vi "API VI Generation tester.vi"() -> ()   [LabVIEW 2020, in "Method Generation.lvlib" / "API VI Generator.lvclass"]
uses:
  API VI Generator.lvclass
  API VI Generator.lvclass/API VI Generator.ctl
panel:
  out "error out":errorcluster
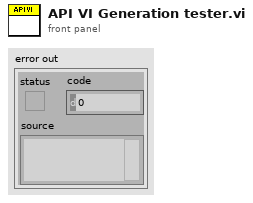
[diagram p1: front panel]
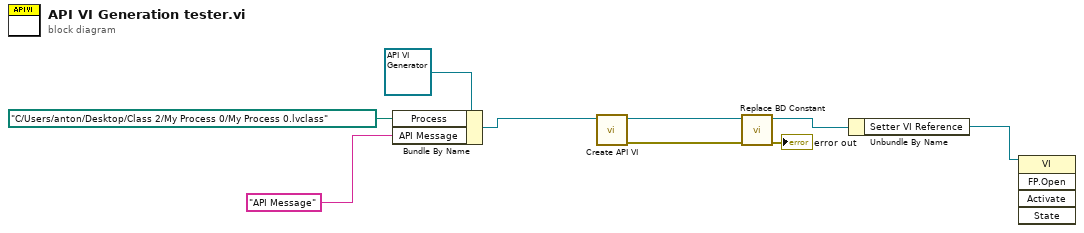
[diagram p0: block diagram]
diagram:
  n1 = Bundle By Name(cluster=refnum<class "API VI Generator.lvclass"> refnum ("New Getter Dialog In"), "Process"=path "C:/Users/anton/Desktop/Class 2/My Process 0/My Process 0.lvclass", "API Message"="API Message" ("Attribute Name")) -> (w8:refnum<class "API VI Generator.lvclass">)
  n2 = call "Create API VI.vi"("Setter Generator In"=w8) -> ("error out"=w1:errorcluster, "Setter Generator Out"=w2:refnum<class "API VI Generator.lvclass">)  [unwired: 9 in]
  n3 = call "Replace BD Constant.vi"("error in (no error)"=w1, "Setter Generator In"=w2) -> ("error out"=→"error out":errorcluster, "Setter Generator Out"=w5:refnum<class "API VI Generator.lvclass">)  [unwired: 8 in]
  n4 = Unbundle By Name(w5) -> ("Setter VI Reference"=w6:refnum<vi>)
  n5 = invoke class="VI" method="FP.Open"(reference=w6) -> ()  [unwired: 4 in, 5 out]
